vi "predict_focus.vi"(3 "Known Y":dbl, 4 "Known X":dbl, 5 "Prediction order":i16=1 min=0 max=2, 6 "focal map fileref":refnum<file>) -> (0 "linear fit return val":i32, 1 "Standard deviation of errors":dbl, 2 "predicted focal position":dbl)   [LabVIEW 2011]
uses:
  <vilib>/Utility/file.llb/Read From Spreadsheet File (DBL).vi
  <vilib>/Analysis/NI_AALPro.lvlib
panel:
  out "input data":dbl[][](array[numeric])
  out "Coefficients":dbl[](array[numeric]) format="%.3e"
  out "MSE":dbl format="%.5f"
  out "Best Fit Z":dbl[](array[numeric]) format="%.2f"
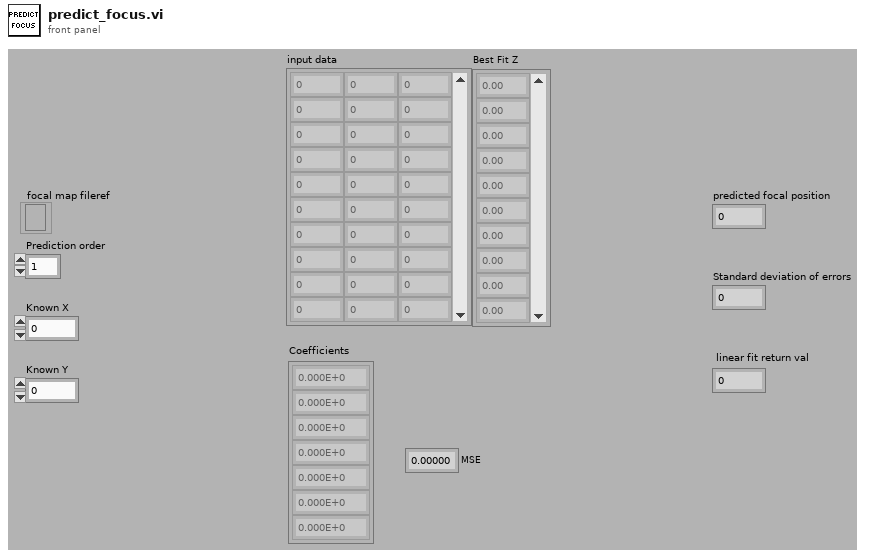
[diagram p1: front panel]
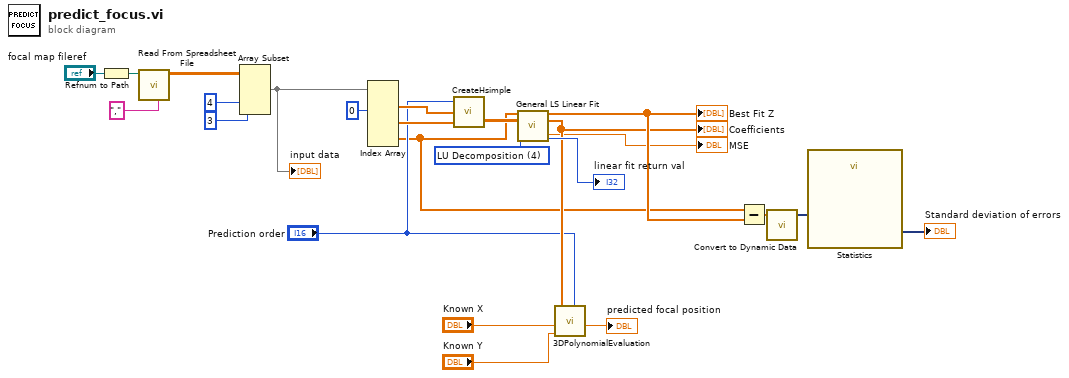
[diagram p0: block diagram]
diagram:
  w6 = u16 4 items=["SVD", "Givens", "Givens2", "Householder", "LU Decomposition", "Cholesky", "SVD for Rank Deficient H"] ("algorithm")
  n1 = Refnum to Path(1:"focal map fileref") -> (0:w1:path)
  n2 = call-poly <vilib>:"Read From Spreadsheet File.vi"("delimiter (\\t)"="," ("delimiter (\\t)"), "file path (dialog if empty)"=w1) -> ("all rows"=w4:dbl[][])  [unwired: 5 in, 4 out]
  n3 = Array Subset(array=w4, index (col)=4 ("index"), length (col)=3 ("length")) -> (w16:dbl[][])  [unwired: 2 in]
  "input data" <- w16
  n4 = Index Array(array=w16, index (col) #1=0 ("disabled index (col)")) -> (element #1=w18:dbl[], element #2=w19:dbl[], element #3=w3:dbl[])  [unwired: 5 in]
  n5 = call "CreateHsimple.vi"("[Y]"=w19, "[X]"=w18, "Highest order"="Prediction order") -> ("H"=w7:dbl[][])  [unwired: 1 in]
  n6 = call <vilib>:"General LS Linear Fit.vi"("Y"=w3, "H"=w7, "algorithm"=w6) -> ("Best Fit"=w20:dbl[], "Coefficients"=w10:dbl[], "mse"=→"MSE":dbl, "error"=→"linear fit return val":i32)  [unwired: 8 in, 1 out]
  "Coefficients" <- w10
  "Best Fit Z" <- w20
  n7 = call "3DPolynomialEvaluation.vi"("y (0.66)"="Known Y", "x (0.34)"="Known X", "a00, a10, a01, ...."=w10, "order (3)"="Prediction order") -> ("z"=→"predicted focal position":dbl)  [unwired: 7 in]
  n8 = Subtract(x=w3, y=w20) -> (x-y=w23:dbl[])
  n9 = call "Convert to Dynamic Data"("Array"=w23) -> ("Dynamic Data Type"=w21:dynamicdata)  [unwired: 3 in]
  n10 = call "Statistics"("Signals"=w21) -> ("Standard Dev"=→"Standard deviation of errors":dynamicdata)  [unwired: 25 in, 1 out]
